vi "Delete Test Names Log File.vi"(10 "name or relative path":string, 11 "file path (use dialog)":path=path "C:/SSP/Snap-On_GEP/trunk/Software/Log Results/TEST NAMES LOG.csv") -> (3 "appended path":path)   [LabVIEW 2015]
uses:
  Test Result.ctl
panel:
  in  "Results":T1[](array[typedef])=[{"StepName"="Test Date", "Status"=FALSE, "Data"="", "Limits"=variant}, {"StepName"="Time", "Status"=FALSE, "Data"="", "Limits"=variant}, {"StepName"="SN", "Status"=FALSE, "Data"="", "Limits"=variant}, {"StepName"="Station ID", "Status"=FALSE, "Data"="", "Limits"=variant}, {"StepName"="Overall Pass/Fail Results", "Status"=FALSE, "Data"="", "Limits"=variant}]
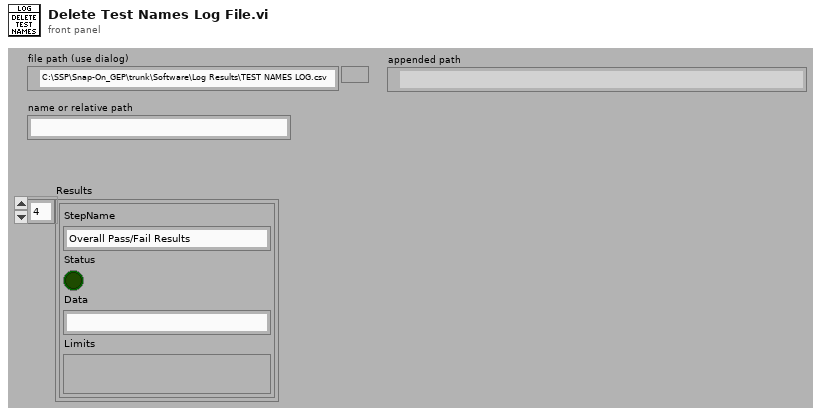
[diagram p1: front panel]
types:
  T1 = typedef "Test Result.ctl" = cluster{"StepName":string, "Status":bool, "Data":string, "Limits":variant}
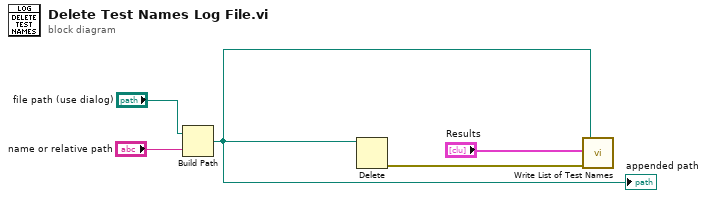
[diagram p0: block diagram]
diagram:
  n1 = Build Path(base path="file path (use dialog)", name or relative path="name or relative path") -> (appended path=w1:path)
  "appended path" <- w1
  n2 = Delete(path (use dialog)=w1) -> (error out=w5:errorcluster)  [unwired: 4 in, 2 out]
  n3 = call "Write List of Test Names.vi"("Results"="Results", "error in (no error)"=w5, "file path (use dialog)"=w1) -> ()  [unwired: 16 in, 1 out]
